vi "Test shm accept Command set Simulation Mode LV.vi"(8 "error in (no error)":errorcluster, 11 "command_setSimulationMode_Ctl":cluster{"mode":i32}) -> (0 "error out":errorcluster, 2 "function return":i32, 3 "command_setSimulationMode_Ctl out":cluster{"mode":i32})   [LabVIEW 2018, in "SALLV_Test.lvlib"]
doc: "int Test_shm_acceptCommand_setSimulationModeLV(Test_command_setSimulationModeLV *command_setSimulationMode_Ctl );"
uses:
  SALLV_Test.lvlib
  SALLV_Test.so
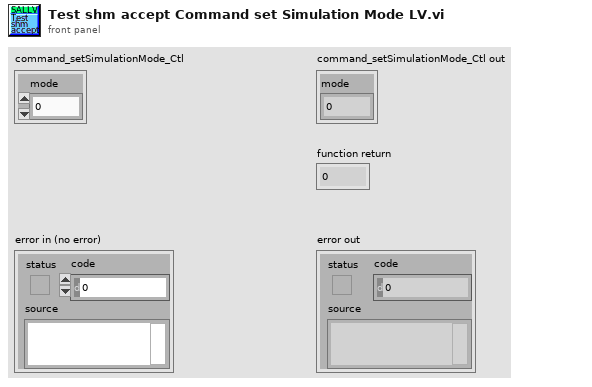
[diagram p1: front panel]
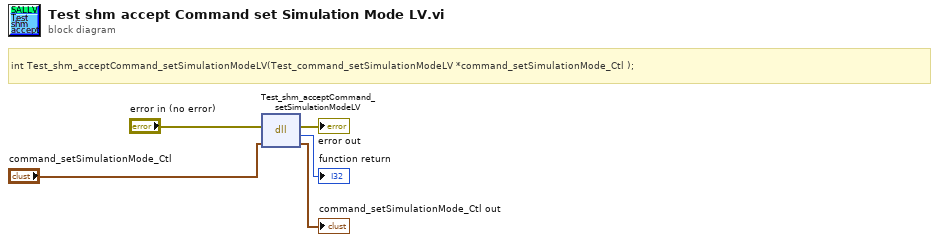
[diagram p0: block diagram]
diagram:
  # "int Test_shm_acceptCommand_setSimulationModeLV(Test_command_setSimulationModeLV *command_setSimulationMode_Ctl );"
  n1 = dll-call lib="home/ttsai/Documents/salLabVIEWtestData/SALLV_Test.*" fn="Test_shm_acceptCommand_setSimulationModeLV"(error in="error in (no error)", "command_setSimulationMode_Ctl"="command_setSimulationMode_Ctl") -> (error out=→"error out":errorcluster, →"function return":i32, "command_setSimulationMode_Ctl"=→"command_setSimulationMode_Ctl out":cluster{"mode":i32})  [unwired: 2 in, 1 out]
